vi "Get New Level.vi"(8 "error in (no error)":errorcluster, 11 "Cooler in":refnum<class "Cooler.lvclass">) -> (0 "error out":errorcluster, 2 "Level":dbl, 3 "Cooler out":refnum<class "Cooler.lvclass">)   [LabVIEW 2012, in "Cooler.lvlib" / "Cooler.lvclass"]
uses:
  Cooler.lvclass
  Cooler.lvclass/Cooler.ctl
  Cooler UI/Cooler UI with Events Messages/Update Temperature Msg/Update Temperature Msg.lvclass/Update Temperature Msg.ctl
  <vilib>/ActorFramework/Message Enqueuer/Message Enqueuer.lvclass/Message Enqueuer.ctl
  <vilib>/ActorFramework/Message Enqueuer/Enqueue.vi
  Simulation/Simulation Data_Global.vi
  <vilib>/ActorFramework/Message Priority Queue/Priority Enqueue.vi
  Cooler UI/Cooler UI with Events Messages/Update Temperature Msg/Update Temperature Msg.lvclass
  Simulation/Simulation.lvlib
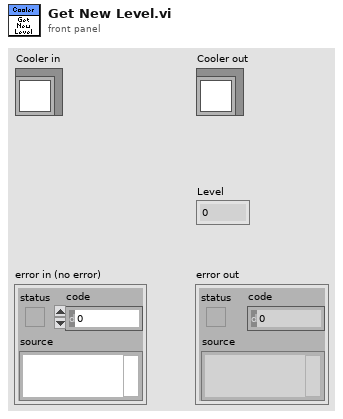
[diagram p1: front panel]
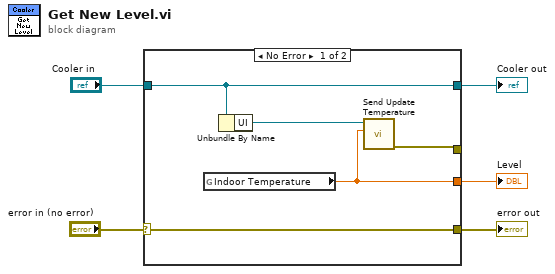
[diagram p0: block diagram]
diagram:
  n1 = case shown="No Error" "error in (no error)" {
    selector: "error in (no error)" -> [w10 _]
    tunnel: "Cooler in" -> [w8 w11]
    tunnel: [w9 _] -> w4
    tunnel: [w8 w11] -> w3
    tunnel: [w10 _] -> w1
    tunnel: [w6 _] -> _
    frame No Error {
      n2 = global read "Simulation Data_Global.vi" "Indoor Temperature"() -> (w9:dbl)
      n3 = Unbundle By Name(w8) -> ("UI"=w7:refnum<class "Message Enqueuer.lvclass">)
      n4 = call "Send Update Temperature.vi"("Temperature"=w9, "Message Enqueuer"=w7) -> ("error out"=w6:errorcluster)  [unwired: 8 in, 1 out]
    }
    frame Error {
    }
  }
  "error out" <- w1
  "Cooler out" <- w3
  "Level" <- w4
